vi "RESPALDO2.vi"() -> ()   [LabVIEW 2017]
uses:
  <vilib>/myRIO/Instrument Drivers/Onboard IO/PWM/typedefs/PWM Reference.ctl
  <vilib>/myRIO/Common/Instrument Driver Framework/Utilities/typedefs/myRIO Generic Hardware Reference.ctl
  <vilib>/myRIO/Common/Instrument Driver Framework/Utilities/typedefs/Hardware Version Enum.ctl
  <vilib>/myRIO/Common/Instrument Driver Framework/Utilities/typedefs/myRIO v1.0 Reference.ctl
  <vilib>/myRIO/Common/Instrument Driver Framework/Utilities/typedefs/Generic FPGA Reference.ctl
  <vilib>/myRIO/Common/Instrument Driver Framework/myRIO v1.0/PWM/typedefs/PWM Channels Enum.ctl
  <vilib>/myRIO/Instrument Drivers/Onboard IO/PWM/typedefs/PWM Configuration.ctl
  <vilib>/userdefined/High Color/nirio_resource_hc.ctl
  <vilib>/myRIO/Instrument Drivers/Onboard IO/DIO/typedefs/DIO Reference.ctl
  <vilib>/myRIO/Common/Instrument Driver Framework/myRIO v1.0/DIO/typedefs/DIO Channels List.ctl
  <vilib>/myRIO/Common/Instrument Driver Framework/myRIO v1.0/DIO/typedefs/DIO Channels Enum.ctl
  <vilib>/myRIO/Common/Instrument Driver Framework/Utilities/vis/Is FPGA Ref Available.vi
  <vilib>/myRIO/Common/Instrument Driver Framework/myRIO v1.0/DIO/vis/myRIO v1.1 Open DIO.vi
  <vilib>/myRIO/Instrument Drivers/Onboard IO/DIO/vis/Write.vi
  <vilib>/myRIO/Common/Instrument Driver Framework/myRIO v1.0/PWM/vis/myRIO v1.1 Open PWM.vi
  <vilib>/myRIO/Common/Instrument Driver Framework/myRIO v1.0/UART/vis/myRIO v1.0 Close UART.vi
  <vilib>/myRIO/Common/Instrument Driver Framework/Utilities/vis/Validate Channels.vi
  <vilib>/myRIO/Common/Instrument Driver Framework/myRIO v1.0/DIO/vis/myRIO v1.0 Reserve DIO.vi
  <vilib>/myRIO/Common/Instrument Driver Framework/myRIO v1.0/PWM/vis/myRIO v1.0 Reserve PWM.vi
  <vilib>/myRIO/Common/Instrument Driver Framework/myRIO v1.0/Resource Manager/vis/myRIO v1.0 Reserve Channel List.vi
  <vilib>/myRIO/Common/Instrument Driver Framework/myRIO v1.0/DIO/vis/myRIO v1.0 Build MUX Configuration DIO.vi
  <vilib>/myRIO/Common/Instrument Driver Framework/myRIO v1.0/PWM/vis/myRIO v1.0 Build MUX Configuration PWM.vi
  <vilib>/myRIO/Common/Instrument Driver Framework/myRIO v1.0/Resource Manager/vis/myRIO v1.0 Reserve Channel.vi
  <vilib>/myRIO/Common/Instrument Driver Framework/myRIO v1.0/Resource Manager/vis/myRIO v1.0 Unreserve Channel.vi
  <vilib>/myRIO/Common/Instrument Driver Framework/myRIO v1.0/Resource Manager/vis/myRIO v1.0 Create Configuration List.vi
  <vilib>/myRIO/Common/Instrument Driver Framework/myRIO v1.0/Resource Manager/vis/myRIO v1.0 Build Mutex Name.vi
  <vilib>/Utility/VariantDataType/GetNumericInfo.vi
  <vilib>/Utility/error.llb/Error Cluster From Error Code.vi
  <vilib>/myRIO/Common/Instrument Driver Framework/myRIO v1.0/myRIO v1.1 Open.vi
  <vilib>/myRIO/Common/Instrument Driver Framework/Utilities/vis/IO Manager.vi
  <vilib>/myRIO/Common/Instrument Driver Framework/Utilities/vis/Configuration Manager.vi
  <vilib>/myRIO/Common/Instrument Driver Framework/myRIO v1.0/Resource Manager/vis/myRIO v1.0 Configure IO.vi
  <vilib>/myRIO/Common/Instrument Driver Framework/myRIO v1.0/myRIO v1.0 Close.vi
  <vilib>/myRIO/Common/Instrument Driver Framework/myRIO v1.0/PWM/vis/myRIO v1.0 Write PWM.vi
  <vilib>/myRIO/Common/Instrument Driver Framework/myRIO v1.0/DIO/vis/myRIO v1.0 Write DIO.vi
  <vilib>/myRIO/Common/Instrument Driver Framework/Utilities/vis/FPGA Ref Manager.vi
  <vilib>/myRIO/Common/Instrument Driver Framework/myRIO v1.0/myRIO v1.0 Reset FPGA.vi
  <vilib>/myRIO/Common/Instrument Driver Framework/myRIO v1.0/IRQ/vis/myRIO v1.0 IRQ Info FGV.vi
  <vilib>/myRIO/Common/Instrument Driver Framework/myRIO v1.0/IRQ/vis/myRIO v1.0 Timer IRQ Info FGV.vi
  <vilib>/myRIO/Common/Instrument Driver Framework/myRIO v1.0/IRQ/vis/myRIO v1.0 ISR Agent.vi
  <vilib>/myRIO/Express VI/Onboard IO/PWM/PWM Express VI.xnode
  <vilib>/myRIO/Instrument Drivers/Onboard IO/PWM/vis/myRIO PWM Open.xnode
  <vilib>/myRIO/Express VI/Onboard IO/DO/DO Express VI.xnode
  <vilib>/myRIO/Instrument Drivers/Onboard IO/DIO/vis/myRIO DIO Open.xnode
  <vilib>/myRIO/Instrument Drivers/Utilities/Utilities.lvlib
  <vilib>/myRIO/Instrument Drivers/Onboard IO/PWM/PWM.lvlib
  <vilib>/myRIO/Instrument Drivers/Onboard IO/DIO/DIO.lvlib
panel:
  out "Numeric 4":dbl
  out "Numeric 3":dbl
  in  "MODO JOG":bool
  out "Numeric 2":dbl
  out "Slide 2":dbl(slide) scale=-200.0..100.0
  out "Slide":dbl(slide) scale=-200.0..100.0
  out "Numeric":dbl
  in  "control":T1(tab)
  in  "PARADA":bool
  out "ESTADO":string
  in  "?":bool
  out "MODO":string
  in  "Boolean":bool
  in  "PWM channel":tag="B/PWM0"
  in  "PWM channel 2":tag="B/PWM0"
  out "offset [%FS] 3":dbl
  in  "null offset 3":bool
  out "duty cycle [%] 3":dbl
  out "pulse width [ms] 3":dbl=1.5
  in  "position 2":dbl(slide) scale=-200.0..200.0
  in  "PWM channel 3":tag="B/PWM0"
  out "offset [%FS] 4":dbl
  in  "null offset 4":bool
  out "duty cycle [%] 4":dbl
  out "pulse width [ms] 4":dbl=1.5
  in  "position [%FS] 4":dbl(slide) scale=-200.0..200.0
  out "offset [%FS] 5":dbl
  in  "null offset 5":bool
  out "duty cycle [%] 5":dbl
  out "pulse width [ms] 5":dbl=1.5
  in  "position [%FS] 5":dbl(slide) scale=-200.0..200.0
  out "position [%FS]":dbl
  out "position [3":dbl
  out "position1":dbl
  out "ventosa":bool
  out "POSICION1":dbl
  out "POSICION2":dbl
  out "POSICION3":dbl
  in  "velocidad":dbl(knob) scale=20.0..250.0
  in  "PARADA":bool
  out "INDICADOR 2":bool
  out "INDICADOR1":bool
  in  "PARADA":bool
  in  ".":dbl(slide) scale=0.0..10.0
  in  ".":dbl(slide) scale=0.0..10.0
  out "String":string
  out "CADENA1":dbl
  out "CADENA2":dbl
  in  "Puero de servicio remoto":u16
  in  "direccion":string
  in  "PARADA":bool
  out "Datos recibidos vía TCP":cluster{dbl, dbl}(graph)
  out "offset [%FS] 2":dbl
  in  "null offset 2":bool
  out "duty cycle [%] 2":dbl
  out "pulse width [ms] 2":dbl=1.5
  in  "freq [Hz] 2":dbl=50.0
  in  "position [%FS] 3":dbl(slide) scale=-400.0..400.0
  in  "PWM channel 6":tag="B/PWM0"
  in  "PWM channel 5":tag="B/PWM0"
  in  "position [%FS] 2":dbl(slide) scale=-400.0..400.0
  in  "freq [Hz]":dbl=50.0
  out "pulse width [ms]":dbl=1.5
  out "duty cycle [%]":dbl
  in  "null offset":bool
  out "offset [%FS]":dbl
  out "offset [%FS] 6":dbl
  in  "null offset 6":bool
  out "duty cycle [%] 6":dbl
  out "pulse width [ms] 6":dbl=1.5
  in  "freq [Hz] 3":dbl=50.0
  in  "position [%FS] 6":dbl(slide) scale=-400.0..400.0
  in  "PWM channel 7":tag="B/PWM0"
  in  "VALVULA":bool
  in  "VELOCIDAD1":dbl(knob) scale=0.0..1.0
  in  "VELOCIDAD 2":dbl(knob) scale=0.0..1.0
  in  "DIRECCION1":bool
  in  "DIRECCION 2":bool
  in  "servomotores":bool
  out "V1":dbl
  out "V2":dbl
  # "BIENVENIDOS A LA\nINTERFAZ DE CONTROL ROBOT DELTA"
  # "INICIO DE PROCESO"
  # "SISTEMA DE ESTADO DE ROBOT DELTA"
  # "SERVOMOTOR1"
  # "SERVOMOTOR2"
  # "SERVOMOTOR3"
  # "VISUALIZACION DE CINTAS TRANSPORTADORAS"
  # "CINTA TRANSPORTADORA1"
  # "CINTA TRANSPORTADORA2"
  # "COMUNICACION CON EL SISTEMA DE VISION"
  # "DATOS DE COMIUNICACION"
  # "VISUALIZACION DE POSCICION"
  # "SERVOMOTOR1"
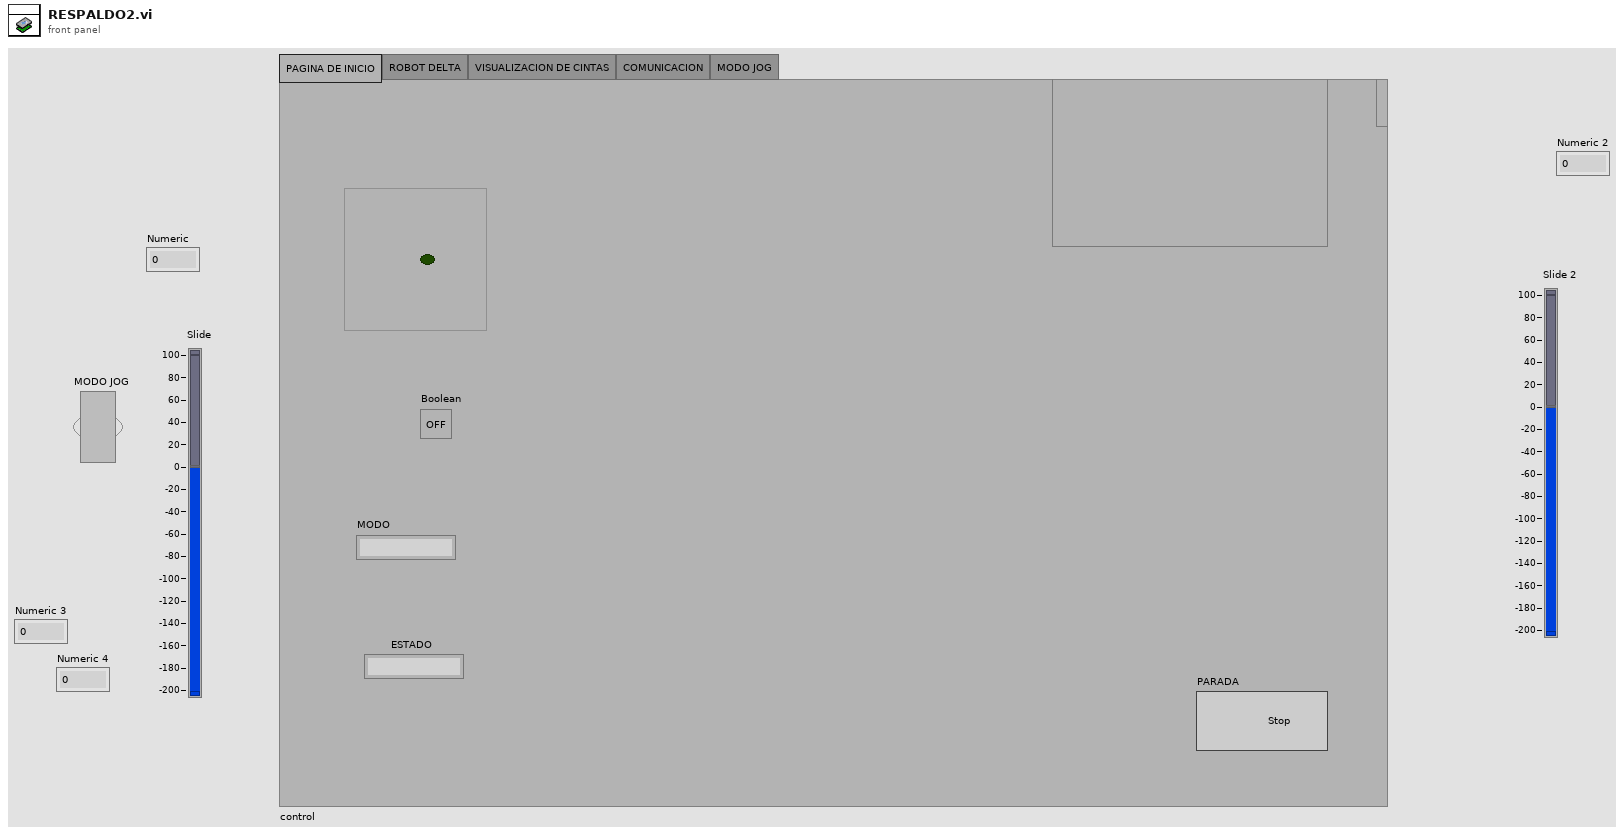
[diagram p1: front panel]
types:
  T1 = enum32{"PAGINA DE INICIO", "ROBOT DELTA", "VISUALIZACION DE CINTAS", "COMUNICACION", "MODO JOG"}
  T2 = enum16{"", "INICIO", "STOP", "DETECCION", "ESPERA", "MOVIMIENTO"}
  T3 = typedef "PWM.lvlib/PWM Reference.ctl" = cluster{"myRIO Reference":T4, "PWM Channels Enum":T8, "PWM Configuration":T9}
  T4 = typedef "myRIO Generic Hardware Reference.ctl" = cluster{"myRIO Model":T5, "myRIO Hardware Reference":T6}
  T5 = typedef "Hardware Version Enum.ctl" = enum16{"Unknown", "myRIO-1900", "myRIO-1950", "roboRIO", "NI ELVIS RIO CM"}
  T6 = typedef "myRIO v1.0 Reference.ctl" = cluster{"Generic FPGA Reference":T7, "Allow multiple opens":bool}
  T7 = typedef "Generic FPGA Reference.ctl" = refnum<k20>
  T8 = typedef "PWM Channels Enum.ctl" = enum16{"Not Connected", "C/PWM0", "C/PWM1", "A/PWM0", "A/PWM1", "A/PWM2", "B/PWM0", "B/PWM1", "B/PWM2", "PWM/PWM0", "PWM/PWM1", "PWM/PWM2", "PWM/PWM3", "PWM/PWM4", "PWM/PWM5", "PWM/PWM6", "PWM/PWM7", "PWM/PWM8", "PWM/PWM9"}
  T9 = typedef "PWM.lvlib/PWM Configuration.ctl" = cluster{"Frequency":dbl, "Duty Cycle":dbl}
  T10 = enum16{"Standard", "Buffered", "CRLF", "Immediate"}
  T11 = typedef "nirio_resource_hc.ctl" = tag
  T12 = typedef "DIO.lvlib/DIO Reference.ctl" = cluster{"myRIO Reference":T4, "DIO Channels List":T13}
  T13 = typedef "DIO Channels List.ctl" = T14[]
  T14 = typedef "DIO Channels Enum.ctl" = enum16{"Not Connected", "C/DIO0", "C/DIO1", "C/DIO2", "C/DIO3", "C/DIO4", "C/DIO5", "C/DIO6", "C/DIO7", "A/DIO0", "A/DIO1", "A/DIO2", "A/DIO3", "A/DIO4", "A/DIO5", "A/DIO6", "A/DIO7", "A/DIO8", "A/DIO9", "A/DIO10", "A/DIO11", "A/DIO12", "A/DIO13", "A/DIO14", "A/DIO15", "B/DIO0", "B/DIO1", "B/DIO2", "B/DIO3", "B/DIO4", "B/DIO5", "B/DIO6", "B/DIO7", "B/DIO8", "B/DIO9", "B/DIO10", "B/DIO11", "B/DIO12", "B/DIO13", "B/DIO14", "B/DIO15", "LED0", "LED1", "LED2", "LED3", "Button0", "DIO/DIO0", "DIO/DIO1", "DIO/DIO2", "DIO/DIO3", "DIO/DIO4", "DIO/DIO5", "DIO/DIO6", "DIO/DIO7", "DIO/DIO8", "DIO/DIO9", "SPI/CS0", "SPI/CS1", "SPI/CS2", "SPI/CS3", "LED RADIO (Green)", "LED RADIO (Red)", "LED COMM (Green)", "LED COMM (Red)", "LED MODE (Green)", "LED MODE (Red)"}
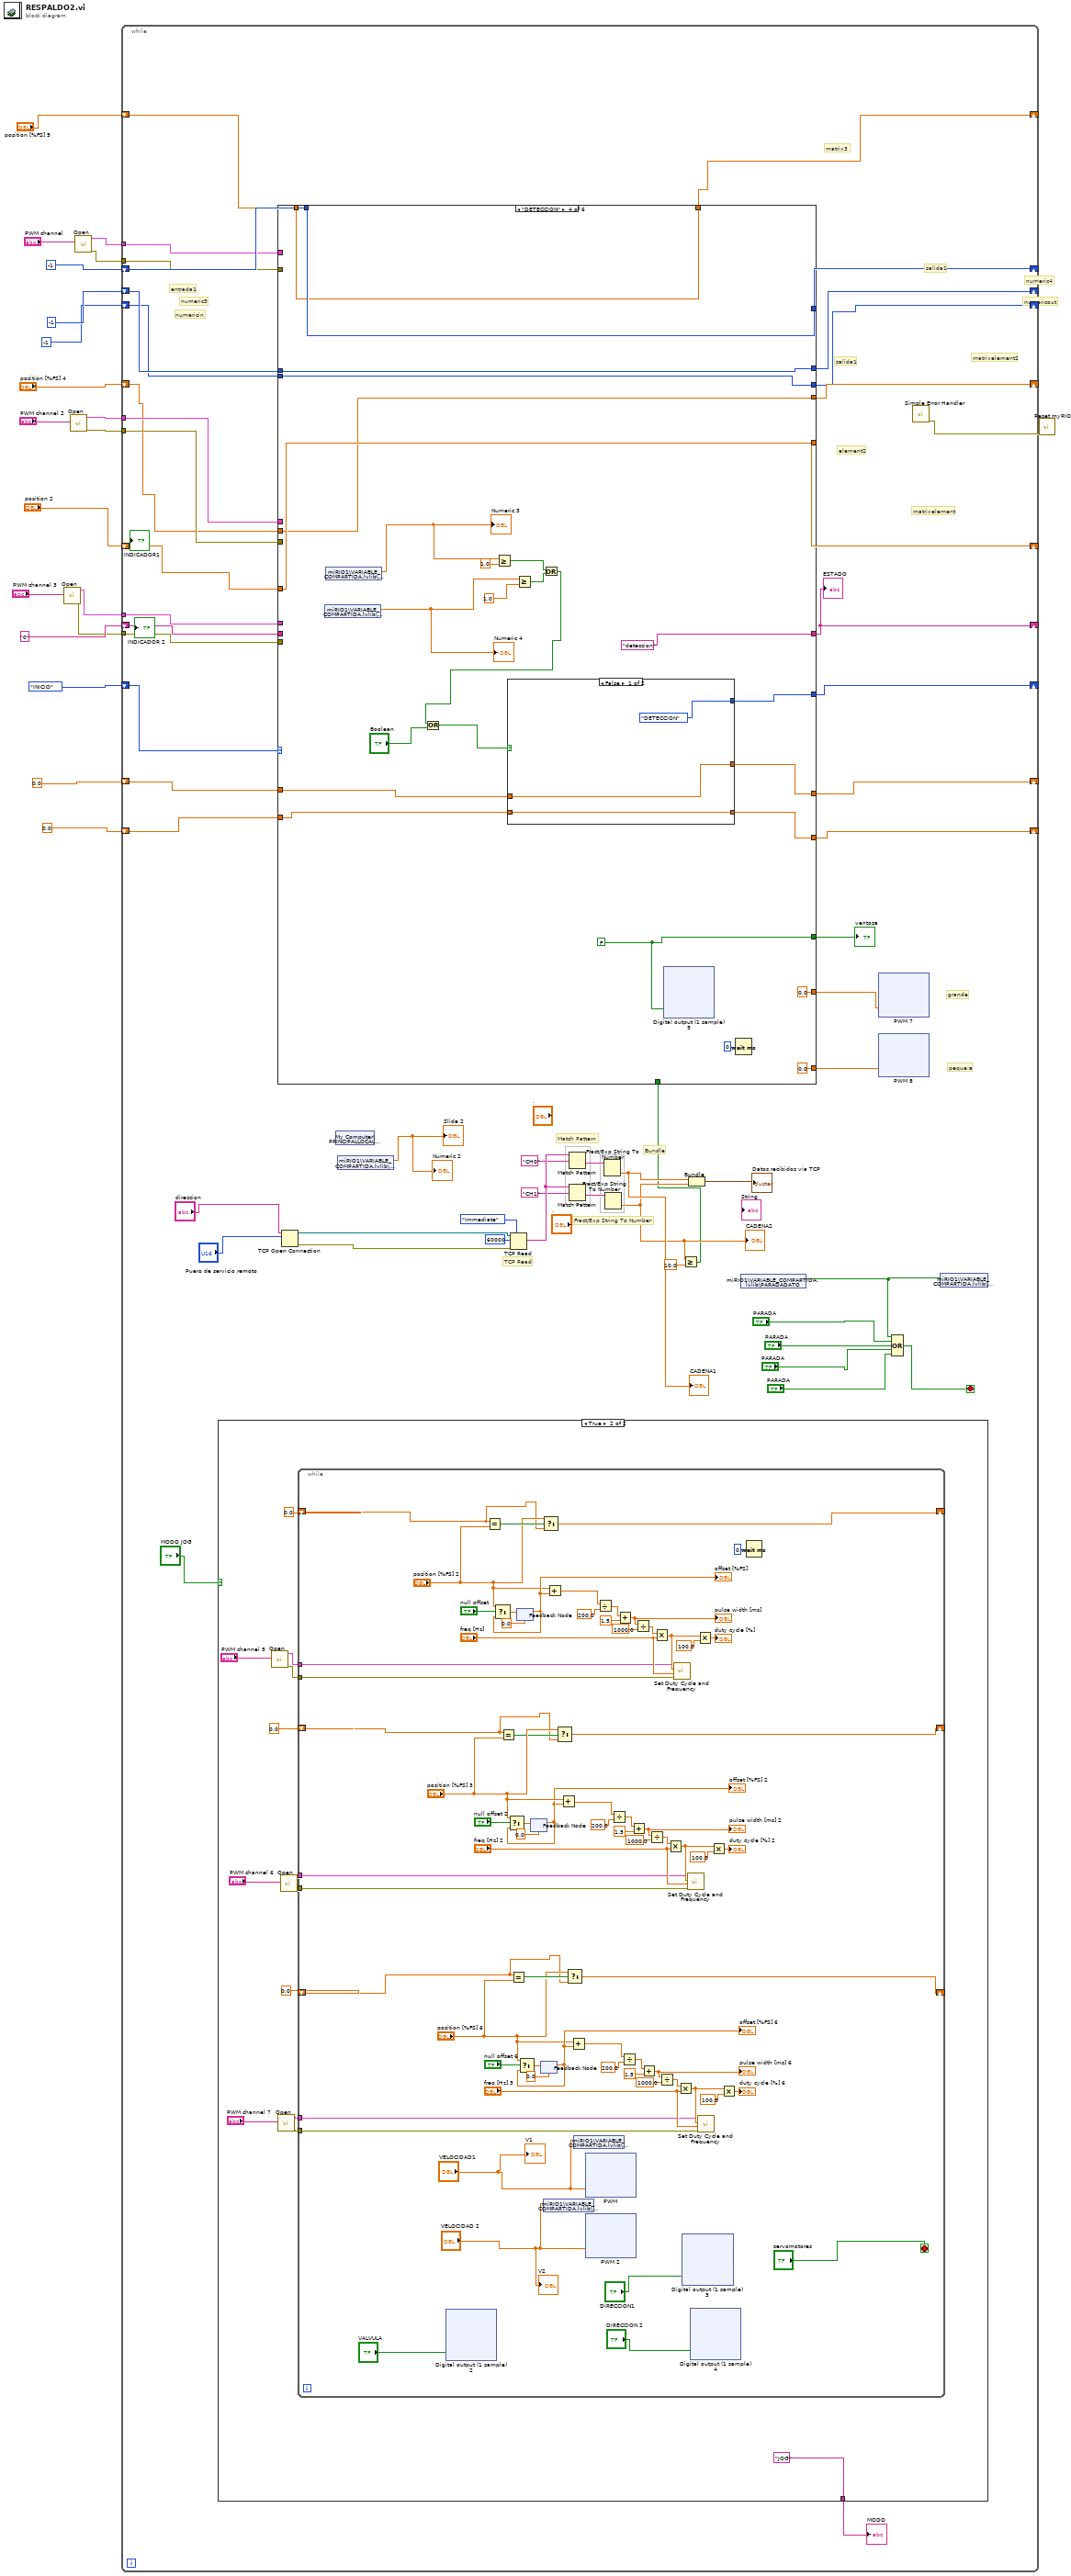
[diagram p0: block diagram]
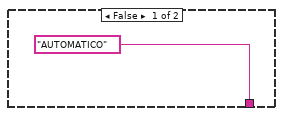
[diagram p2: hidden frame]
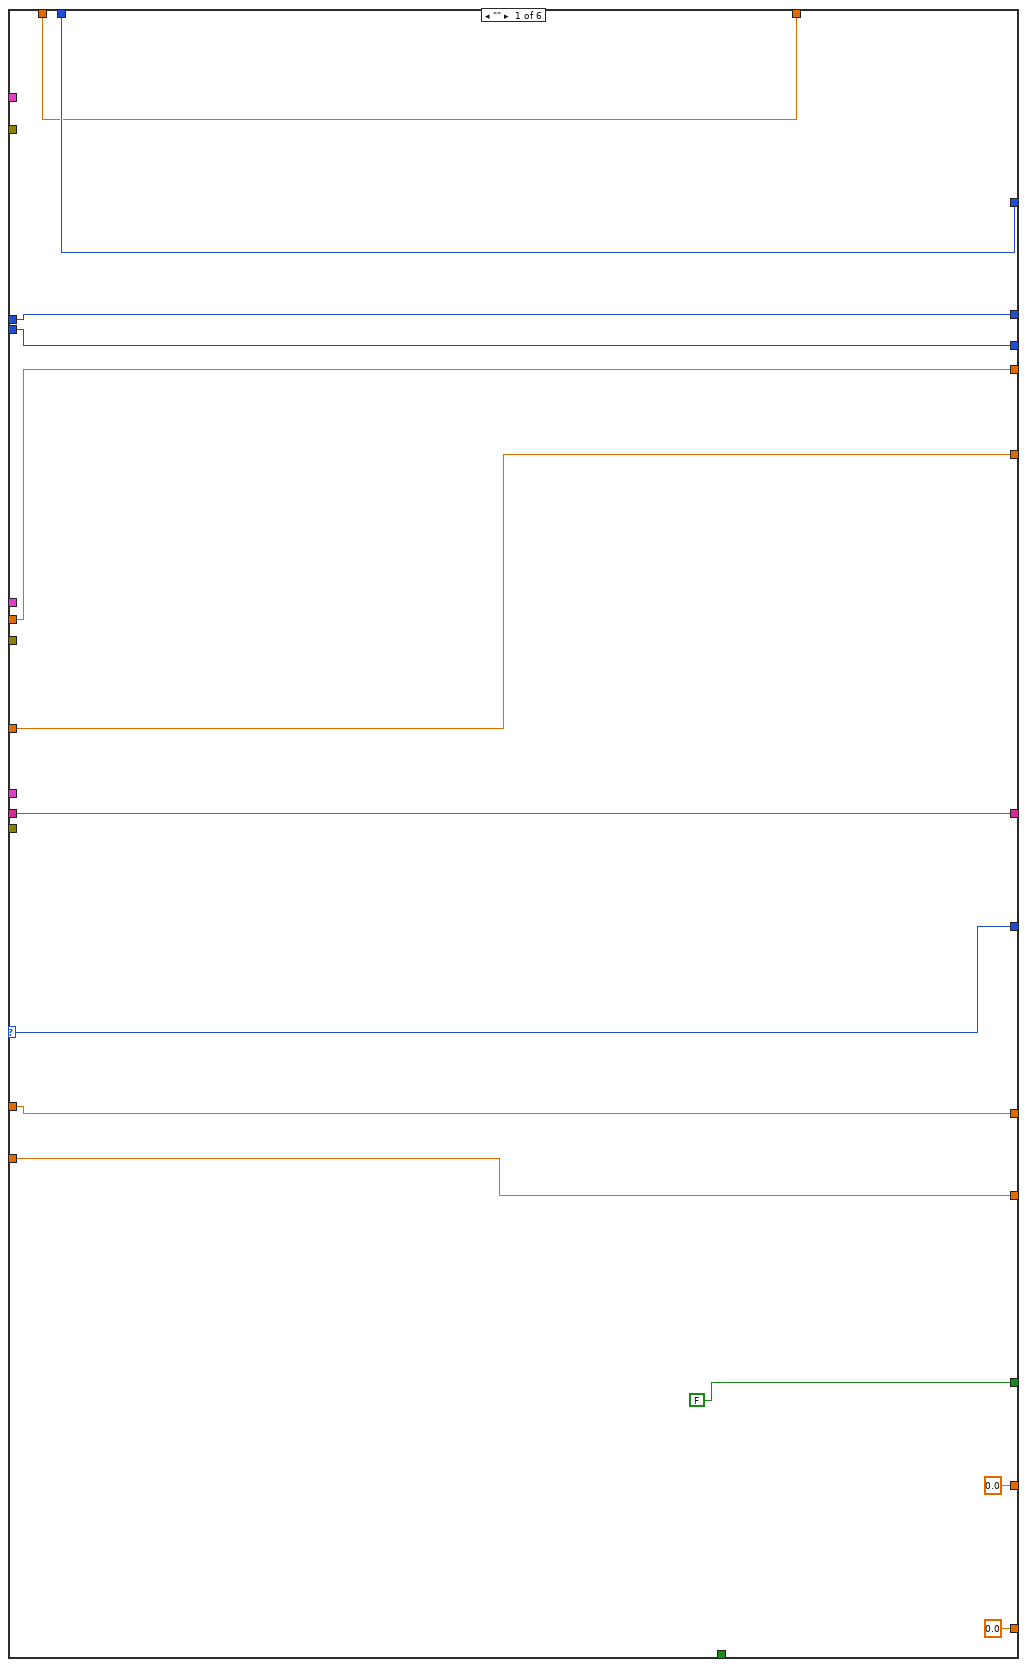
[diagram p3: hidden frame]
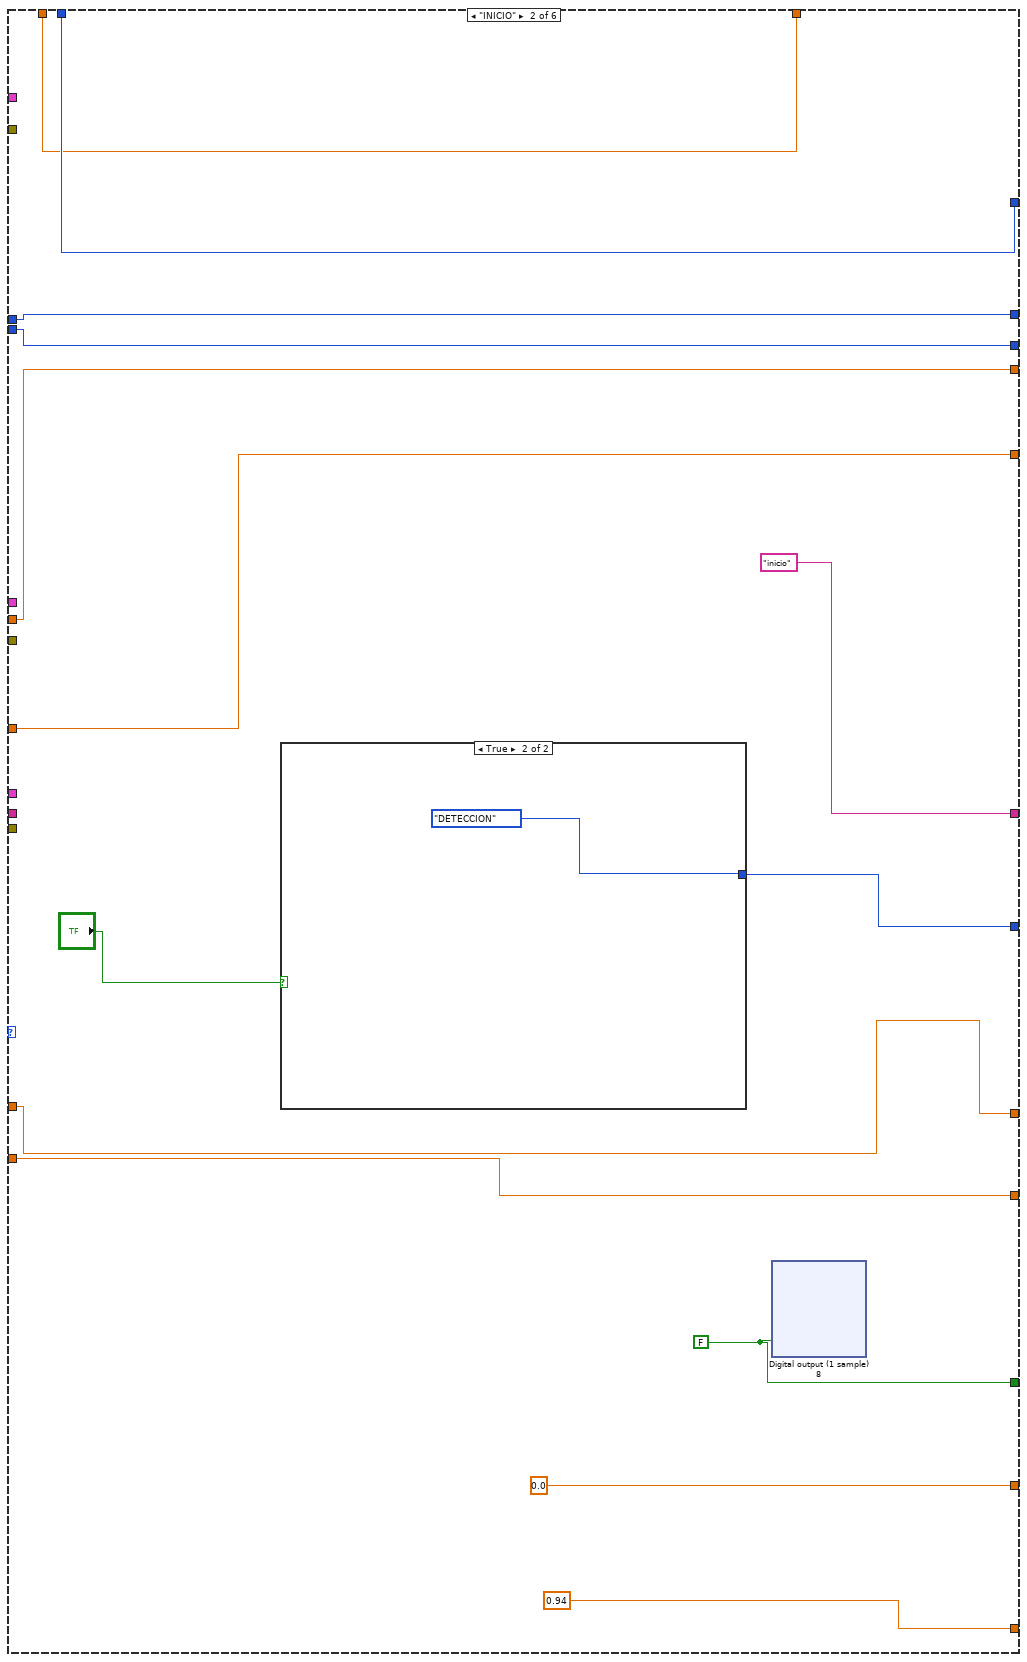
[diagram p4: hidden frame]
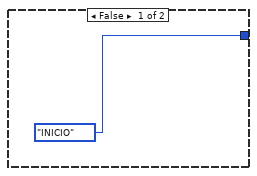
[diagram p5: hidden frame]
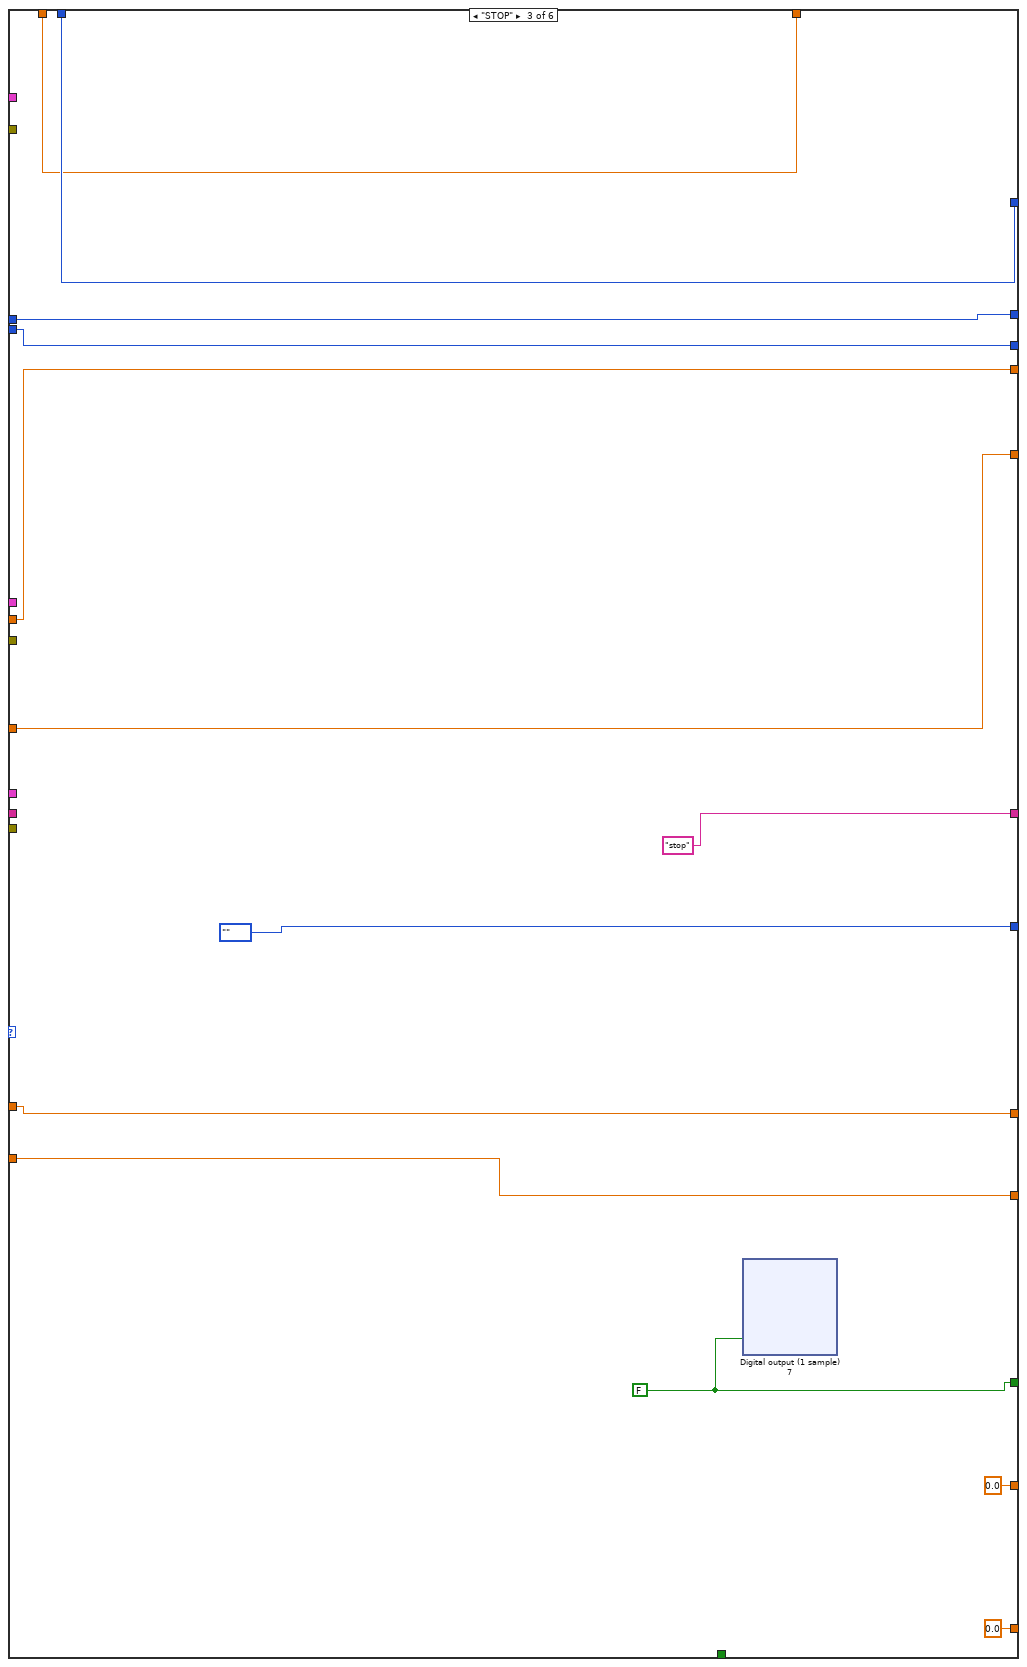
[diagram p6: hidden frame]
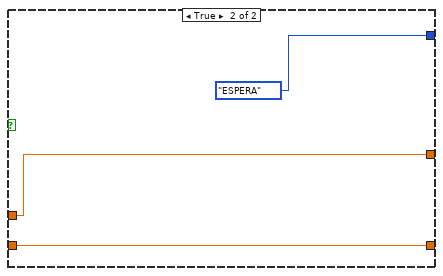
[diagram p7: hidden frame]
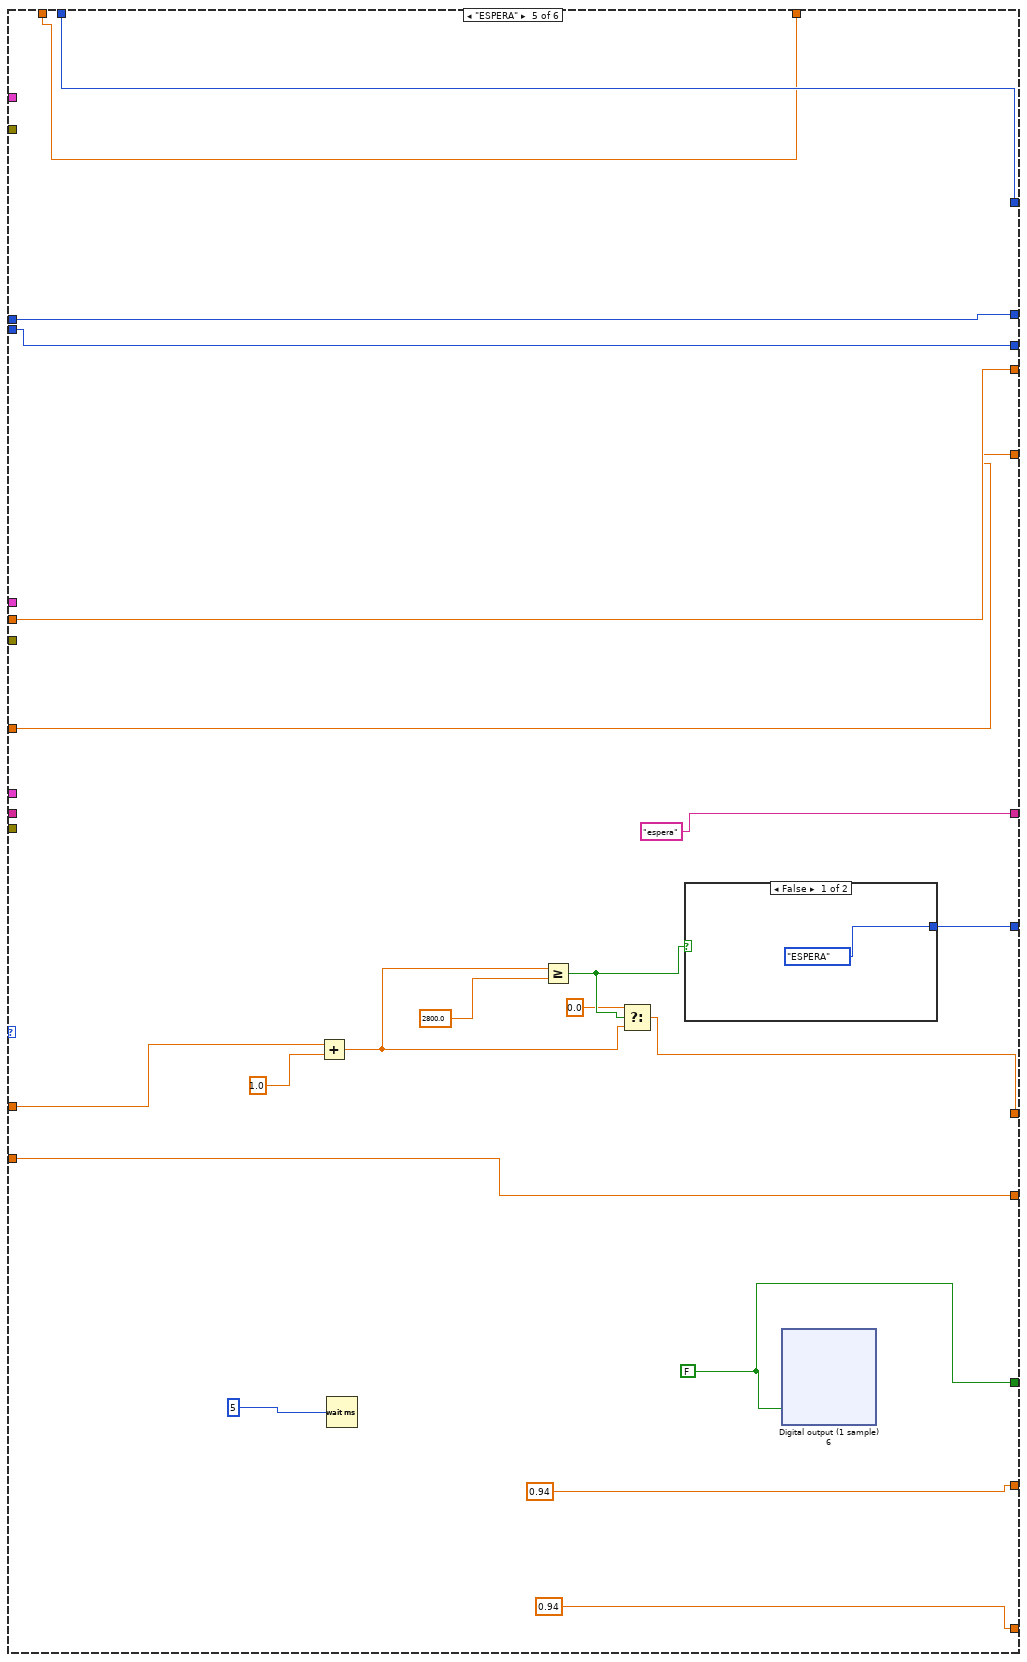
[diagram p8: hidden frame]
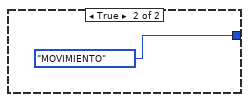
[diagram p9: hidden frame]
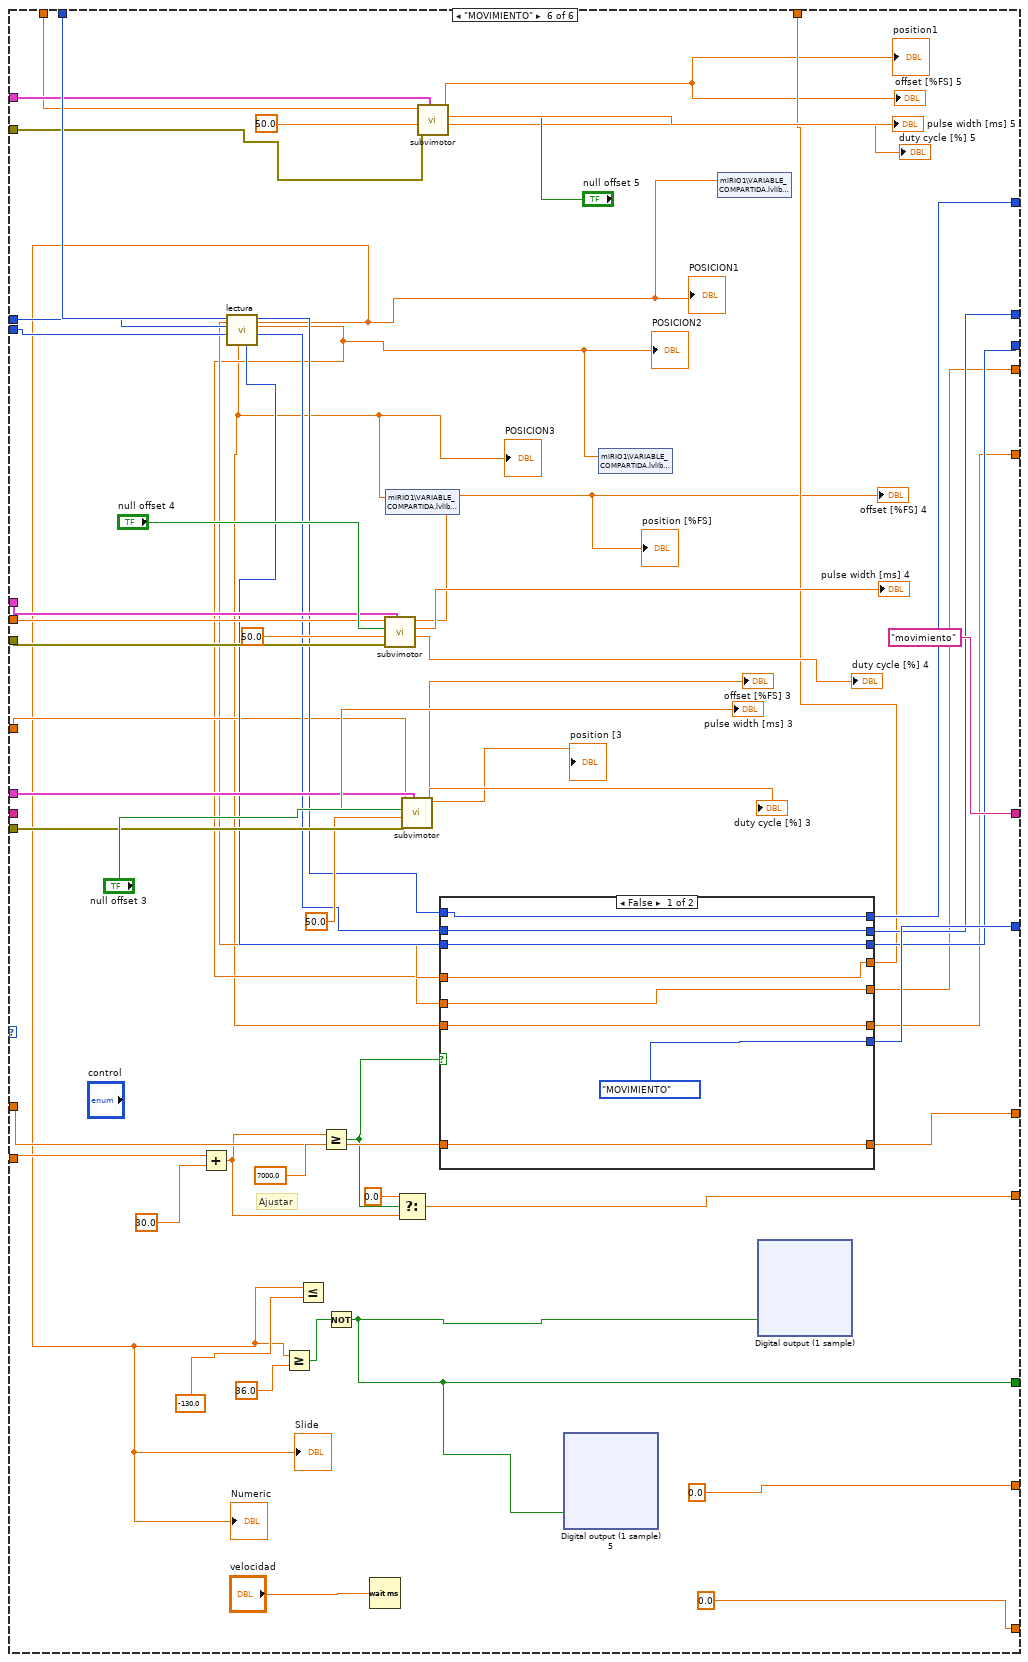
[diagram p10: hidden frame]
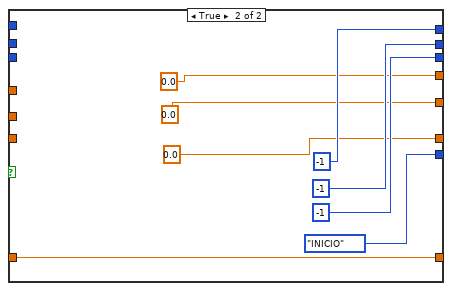
[diagram p11: hidden frame]
diagram:
  # "numericout"
  # "numeric4"
  # "salida1"
  n1 = call <vilib>:"Open.vi"("Channel Name"="PWM channel 3") -> ("error out"=w8:errorcluster, "PWM Ref Out"=w9:T3)  [unwired: 9 in]
  n2 = call <vilib>:"Open.vi"("Channel Name"="PWM channel 2") -> ("error out"=w5:errorcluster, "PWM Ref Out"=w6:T3)  [unwired: 9 in]
  n3 = call <vilib>:"Open.vi"("Channel Name"="PWM channel") -> ("error out"=w2:errorcluster, "PWM Ref Out"=w3:T3)  [unwired: 9 in]
  n4 = while {
    shift-right: [w57] -> _
    shift-left: -1 -> [w61]
    shift-right: [w55] -> _
    shift-left: -1 -> [w60]
    shift-right: [w54] -> _
    shift-left: -1 -> [w59]
    shift-right: [w58] -> _
    shift-left: "position [%FS] 5" -> [w50]
    shift-right: [w56] -> _
    shift-left: "position [%FS] 4" -> [w62]
    shift-right: [w53] -> _
    shift-left: "position 2" -> [w65]
    shift-right: [w73] -> _
    shift-left: T2."INICIO" -> [w74]
    shift-right: [w72] -> _
    shift-left: 0.0 -> [w71]
    shift-right: [w70] -> _
    shift-left: 0.0 -> [w49]
    shift-right: [w69] -> _
    shift-left: "0" ("String") -> [w68]
    tunnel: w9 -> [w67]
    tunnel: w8 -> [w66]
    tunnel: w6 -> [w64]
    tunnel: w5 -> [w63]
    tunnel: w3 -> [w52]
    tunnel: w2 -> [w51]
    stop <- w24 stop-if-true
    # "grande"
    # "peque;a"
    # "matrixelement2"
    # "matrixelement"
    # "Bundle"
    # "TCP Read"
    # "Fract/Exp String To Number"
    # "Match Pattern"
    # "element2"
    # "salida1"
    # "matrix3"
    # "numericin"
    # "numeric3"
    # "entrada1"
    n5 = case shown="True" "MODO JOG" {
      tunnel: ["AUTOMATICO" ("MODO") "JOG" ("MODO")] -> w26
      frame False {
      }
      frame True {
        n6 = call <vilib>:"Open.vi"("Channel Name"="PWM channel 5") -> ("error out"=w156:errorcluster, "PWM Ref Out"=w157:T3)  [unwired: 9 in]
        n7 = call <vilib>:"Open.vi"("Channel Name"="PWM channel 7") -> ("error out"=w150:errorcluster, "PWM Ref Out"=w151:T3)  [unwired: 9 in]
        n8 = call <vilib>:"Open.vi"("Channel Name"="PWM channel 6") -> ("error out"=w153:errorcluster, "PWM Ref Out"=w154:T3)  [unwired: 9 in]
        n9 = while {
          tunnel: w157 -> [w210]
          tunnel: w156 -> [w209]
          shift-right: [w208] -> _
          shift-left: 0.0 ("position [%FS] 2") -> [w207]
          shift-right: [w188] -> _
          shift-left: 0.0 ("position [%FS] 3") -> [w189]
          tunnel: w154 -> [w187]
          tunnel: w153 -> [w186]
          shift-right: [w167] -> _
          shift-left: 0.0 ("position [%FS] 6") -> [w168]
          tunnel: w151 -> [w166]
          tunnel: w150 -> [w165]
          stop <- "servomotores" stop-if-true
          n10 = xnode "Digital output (1 sample) 2"("B/DIO2 (Pin 15)"="VALVULA") -> ()  [unwired: 1 in, 1 out]
          n11 = Equal?(x=w207, y="position [%FS] 2") -> (x = y?=w212:bool)
          n12 = Equal?(x=w189, y="position [%FS] 3") -> (x = y?=w205:bool)
          n13 = Equal?(x=w168, y="position [%FS] 6") -> (x = y?=w170:bool)
          n14 = feedback #1(0.0 ("position [%FS]")) -> (w218:dbl)
          "offset [%FS]" <- w218
          n15 = Select(t="position [%FS] 2", s="null offset", f=w218) -> (s? t:f=w220:dbl)
          n16 = feedback-in #1(w220) -> ()
          n17 = feedback #2(0.0 ("position [%FS]")) -> (w199:dbl)
          "offset [%FS] 2" <- w199
          n18 = Select(t="position [%FS] 3", s="null offset 2", f=w199) -> (s? t:f=w197:dbl)
          n19 = feedback-in #2(w197) -> ()
          n20 = feedback #3(0.0 ("position [%FS]")) -> (w176:dbl)
          "offset [%FS] 6" <- w176
          n21 = Select(t="position [%FS] 6", s="null offset 6", f=w176) -> (s? t:f=w178:dbl)
          n22 = feedback-in #3(w178) -> ()
          n23 = Select(t="position [%FS] 2", s=w212, f=w207) -> (s? t:f=w208:dbl)
          n24 = shared-variable "miRIO1\\VARIABLE_COMPARTIDA.lvlib\\MOTOR2"("VELOCIDAD 2") -> ()  [unwired: 1 in, 1 out]
          n25 = Add(x="position [%FS] 2", y=w218) -> (x+y=w219:dbl)
          n26 = Select(t="position [%FS] 3", s=w205, f=w189) -> (s? t:f=w188:dbl)
          n27 = Add(x="position [%FS] 3", y=w199) -> (x+y=w198:dbl)
          n28 = Select(t="position [%FS] 6", s=w170, f=w168) -> (s? t:f=w167:dbl)
          n29 = Add(x="position [%FS] 6", y=w176) -> (x+y=w177:dbl)
          n30 = shared-variable "miRIO1\\VARIABLE_COMPARTIDA.lvlib\\MOTOR1"("VELOCIDAD1") -> ()  [unwired: 1 in, 1 out]
          n31 = xnode "PWM"("Duty Cycle"="VELOCIDAD1") -> ()  [unwired: 1 in, 1 out]
          n32 = xnode "PWM 2"("Duty Cycle"="VELOCIDAD 2") -> ()  [unwired: 1 in, 1 out]
          n33 = Divide(x=w219, y=200.0) -> (x/y=w226:dbl)
          n34 = Divide(x=w198, y=200.0) -> (x/y=w191:dbl)
          n35 = Add(x=w226, y=1.5) -> (x+y=w224:dbl)
          "pulse width [ms]" <- w224
          n36 = Divide(x=w177, y=200.0) -> (x/y=w184:dbl)
          n37 = Add(x=w191, y=1.5) -> (x+y=w193:dbl)
          "pulse width [ms] 2" <- w193
          n38 = Divide(x=w224, y=1000.0) -> (x/y=w217:dbl)
          n39 = Add(x=w184, y=1.5) -> (x+y=w182:dbl)
          "pulse width [ms] 6" <- w182
          n40 = Divide(x=w193, y=1000.0) -> (x/y=w200:dbl)
          n41 = Multiply(x=w217, y="freq [Hz]") -> (x*y=w214:dbl)
          n42 = Divide(x=w182, y=1000.0) -> (x/y=w175:dbl)
          n43 = Multiply(x=w200, y="freq [Hz] 2") -> (x*y=w203:dbl)
          n44 = call <vilib>:"Set Duty Cycle and Frequency.vi"("error in (no error)"=w209, "Frequency [Hz]"="freq [Hz]", "Duty Cycle"=w214, "PWM Ref In"=w210) -> ()  [unwired: 5 in, 2 out]
          n45 = Multiply(x=w175, y="freq [Hz] 3") -> (x*y=w172:dbl)
          n46 = xnode "Digital output (1 sample) 3"("B/DIO0 (Pin 11)"="DIRECCION1") -> ()  [unwired: 1 in, 1 out]
          n47 = call <vilib>:"Set Duty Cycle and Frequency.vi"("error in (no error)"=w186, "Frequency [Hz]"="freq [Hz] 2", "Duty Cycle"=w203, "PWM Ref In"=w187) -> ()  [unwired: 5 in, 2 out]
          n48 = xnode "Digital output (1 sample) 4"("B/DIO1 (Pin 13)"="DIRECCION 2") -> ()  [unwired: 1 in, 1 out]
          n49 = Multiply(x=w214, y=100.0) -> (x*y=→"duty cycle [%]":dbl)
          n50 = call <vilib>:"Set Duty Cycle and Frequency.vi"("error in (no error)"=w165, "Frequency [Hz]"="freq [Hz] 3", "Duty Cycle"=w172, "PWM Ref In"=w166) -> ()  [unwired: 5 in, 2 out]
          n51 = Multiply(x=w203, y=100.0) -> (x*y=→"duty cycle [%] 2":dbl)
          n52 = Multiply(x=w172, y=100.0) -> (x*y=→"duty cycle [%] 6":dbl)
          n53 = Wait (ms)(milliseconds to wait=u32 0) -> ()  [unwired: 1 out]
          "V1" <- "VELOCIDAD1"
          "V2" <- "VELOCIDAD 2"
        }
      }
    }
    "MODO" <- w26
    n54 = TCP Open Connection(address="direccion", remote port or service name="Puero de servicio remoto") -> (connection ID=w48:refnum<k5>, error out=w47:errorcluster)  [unwired: 3 in]
    n55 = shared-variable "My Computer\\PRINCIPALLOCAL1.lvlib\\POS1"() -> ()  [unwired: 1 in, 2 out]
    n56 = shared-variable "miRIO1\\VARIABLE_COMPARTIDA.lvlib\\POSICION1"() -> (→"Slide 2" →"Numeric 2":dbl)  [unwired: 1 in, 1 out]
    n57 = TCP Read(connection ID=w48, bytes to read=60000, error in (no error)=w47, 7:T10."Immediate" ("mode (standard)")) -> (data out=w44:string)  [unwired: 1 in, 2 out]
    n58 = Match Pattern(string=w44, regular expression="CH0") -> (after substring=w46:string)  [unwired: 1 in, 3 out]
    n59 = Match Pattern(string=w44, regular expression="CH1") -> (after substring=w45:string)  [unwired: 1 in, 3 out]
    n60 = Fract/Exp String To Number(string=w46) -> (number=w42:dbl)  [unwired: 3 in, 1 out]
    "CADENA1" <- w42
    n61 = Fract/Exp String To Number(string=w45) -> (number=w37:dbl)  [unwired: 3 in, 1 out]
    "CADENA2" <- w37
    n62 = Greater Or Equal?(x=w37, y=10.0) -> (x >= y?=w35:bool)
    n63 = case shown="\"DETECCION\"" w74 {
      selector: w74 -> [w416 _ _ _ _ _]
      tunnel: [w416 w430 T2."" w540 w598 w693] -> w73
      tunnel: [w415 w429 w479 w539 w593 w692] -> w72
      tunnel: w71 -> [w415 w429 w479 w538 w600 w691]
      tunnel: [w414 w428 w478 w537 w597 w686] -> w70
      tunnel: w49 -> [w414 w428 w478 w536 w597 w653]
      tunnel: [w413 "inicio" ("String") "stop" ("String") "deteccion" ("String") "espera" ("String") "movimiento" ("String")] -> w69
      tunnel: w68 -> [w413 _ _ _ _ _]
      tunnel: w67 -> [_ _ _ _ _ w682]
      tunnel: w66 -> [_ _ _ _ _ w681]
      tunnel: w65 -> [w408 w421 w471 w530 w586 w652]
      tunnel: w64 -> [_ _ _ _ _ w676]
      tunnel: w63 -> [_ _ _ _ _ w675]
      tunnel: w62 -> [w409 w422 w472 w529 w587 w673]
      tunnel: w61 -> [w412 w426 w476 w534 w589 w672]
      tunnel: w60 -> [w411 w425 w475 w533 w591 w671]
      tunnel: w59 -> [w410 w424 w474 w532 w590 w670]
      tunnel: [w407 w423 w473 w531 w588 w656] -> w58
      tunnel: [w412 w426 w476 w534 w589 w661] -> w57
      tunnel: [w409 w422 w472 w529 w587 w655] -> w56
      tunnel: [w411 w425 w475 w533 w591 w659] -> w55
      tunnel: [w410 w424 w474 w532 w590 w657] -> w54
      tunnel: [w408 w421 w471 w530 w586 w654] -> w53
      tunnel: w52 -> [_ _ _ _ _ w666]
      tunnel: w51 -> [_ _ _ _ _ w665]
      tunnel: w50 -> [w407 w423 w473 w531 w588 w663]
      tunnel: w35 -> [_ _ _ _ _ _]
      tunnel: [FALSE w419 w470 w528 w585 w650] -> w25
      tunnel: [0.0 ("Duty Cycle") 0.94 ("Duty Cycle") 0.0 ("Duty Cycle") 0.0 ("Duty Cycle") 0.94 ("Duty Cycle") 0.0 ("Duty Cycle")] -> w22
      tunnel: [0.0 ("Duty Cycle") 0.0 ("Duty Cycle") 0.0 ("Duty Cycle") 0.0 ("Duty Cycle") 0.94 ("Duty Cycle") 0.0 ("Duty Cycle")] -> w21
      frame "" {
      }
      frame "INICIO" {
        w419 = FALSE ("B/DIO2 (Pin 15)")
        n64 = case shown="True" "?" {
          tunnel: [T2."INICIO" T2."DETECCION"] -> w430
          frame False {
          }
          frame True {
          }
        }
        n65 = xnode "Digital output (1 sample) 8"("B/DIO2 (Pin 15)"=w419) -> ()  [unwired: 1 in, 1 out]
      }
      frame "STOP" {
        w470 = FALSE ("B/DIO2 (Pin 15)")
        n66 = xnode "Digital output (1 sample) 7"("B/DIO2 (Pin 15)"=w470) -> ()  [unwired: 1 in, 1 out]
      }
      frame "DETECCION" {
        w528 = FALSE ("B/DIO2 (Pin 15)")
        n67 = shared-variable "miRIO1\\VARIABLE_COMPARTIDA.lvlib\\POSICION2"() -> (w527:dbl)  [unwired: 1 in, 1 out]
        "Numeric 4" <- w527
        n68 = shared-variable "miRIO1\\VARIABLE_COMPARTIDA.lvlib\\POSICION1"() -> (w526:dbl)  [unwired: 1 in, 1 out]
        "Numeric 3" <- w526
        n69 = Greater Or Equal?(x=w526, y=1.0) -> (x >= y?=w523:bool)
        n70 = Greater Or Equal?(x=w527, y=1.0) -> (x >= y?=w522:bool)
        n71 = Or(x=w523, y=w522) -> (x .or. y?=w519:bool)
        n72 = Or(x=w519, y="Boolean") -> (x .or. y?=w520:bool)
        n73 = case shown="False" w520 {
          tunnel: [T2."DETECCION" T2."ESPERA"] -> w540
          tunnel: [w577 w580] -> w539
          tunnel: w538 -> [w577 w580]
          tunnel: [w576 w579] -> w537
          tunnel: w536 -> [w576 w579]
          frame False {
          }
          frame True {
          }
        }
        n74 = xnode "Digital output (1 sample) 9"("B/DIO2 (Pin 15)"=w528) -> ()  [unwired: 1 in, 1 out]
        n75 = Wait (ms)(milliseconds to wait=u32 0) -> ()  [unwired: 1 out]
      }
      frame "ESPERA" {
        w585 = FALSE ("B/DIO2 (Pin 15)")
        n76 = Add(x=w600, y=1.0) -> (x+y=w594:dbl)
        n77 = Wait (ms)(milliseconds to wait=u32 5) -> ()  [unwired: 1 out]
        n78 = Greater Or Equal?(x=w594, y=2800.0) -> (x >= y?=w595:bool)
        n79 = Select(t=0.0, s=w595, f=w594) -> (s? t:f=w593:dbl)
        n80 = case shown="False" w595 {
          tunnel: [T2."ESPERA" T2."MOVIMIENTO"] -> w598
          frame False {
          }
          frame True {
          }
        }
        n81 = xnode "Digital output (1 sample) 6"("B/DIO2 (Pin 15)"=w585) -> ()  [unwired: 1 in, 1 out]
      }
      frame "MOVIMIENTO" {
        # "Ajustar"
        n82 = Add(x=w653, y=30.0) -> (x+y=w687:dbl)
        n83 = call "lectura.vi"("Numeric in"=w670, "Numeric 3"=w671, "entrada1"=w672) -> ("Numeric 4"=w660:i32, "Real Matrix Element 2"=w643:dbl, "salida1"=w662:i32, "Numeric out"=w658:i32, "Real Matrix Element 3"=w644:dbl, "Real Matrix Element"=w642:dbl)  [unwired: 3 in]
        "POSICION1" <- w644
        "POSICION2" <- w643
        "POSICION3" <- w642
        "Slide" <- w644
        "Numeric" <- w644
        n84 = Greater Or Equal?(x=w644, y=36.0) -> (x >= y?=w648:bool)
        n85 = Less Or Equal?(x=w644, y=-130.0) -> ()  [unwired: 1 out]
        n86 = Greater Or Equal?(x=w687, y=7000.0) -> (x >= y?=w689:bool)
        n87 = Not(x=w648) -> (.not. x?=w650:bool)
        n88 = Wait (ms)(milliseconds to wait="velocidad") -> ()  [unwired: 1 out]
        n89 = call "subvimotor.vi"("PWM Ref Out"=w676, "error in (no error)"=w675, "freq [Hz] 3"=50.0, "null offset 3"="null offset 4", "position [%FS] 3"=w673) -> ("Numeric"=→"duty cycle [%] 4":dbl, "Numeric 2"=→"pulse width [ms] 4":dbl, "position [%FS]"=→"offset [%FS] 4" →"position [%FS]":dbl)  [unwired: 4 in]
        n90 = shared-variable "miRIO1\\VARIABLE_COMPARTIDA.lvlib\\ZPOS"(w642) -> ()  [unwired: 1 in, 1 out]
        n91 = Select(t=0.0, s=w689, f=w687) -> (s? t:f=w686:dbl)
        n92 = call "subvimotor.vi"("PWM Ref Out"=w682, "error in (no error)"=w681, "freq [Hz] 3"=50.0, "null offset 3"="null offset 3", "position [%FS] 3"=w652) -> ("Numeric"=→"duty cycle [%] 3":dbl, "Numeric 2"=→"pulse width [ms] 3":dbl, "position [%FS]"=→"offset [%FS] 3" →"position [3":dbl)  [unwired: 4 in]
        n93 = call "subvimotor.vi"("PWM Ref Out"=w666, "error in (no error)"=w665, "freq [Hz] 3"=50.0, "null offset 3"="null offset 5", "position [%FS] 3"=w663) -> ("Numeric"=→"duty cycle [%] 5":dbl, "Numeric 2"=→"pulse width [ms] 5":dbl, "position [%FS]"=→"offset [%FS] 5" →"position1":dbl)  [unwired: 4 in]
        n94 = case shown="False" w689 {
          tunnel: [T2."MOVIMIENTO" T2."INICIO"] -> w693
          tunnel: [w772 w780] -> w692
          tunnel: w691 -> [w772 w780]
          tunnel: w662 -> [w771 _]
          tunnel: [w771 -1] -> w661
          tunnel: w660 -> [w770 _]
          tunnel: [w770 -1] -> w659
          tunnel: w658 -> [w769 _]
          tunnel: [w769 -1] -> w657
          tunnel: w644 -> [w768 _]
          tunnel: [w768 0.0 ("t")] -> w656
          tunnel: w643 -> [w767 _]
          tunnel: [w767 0.0 ("t")] -> w655
          tunnel: w642 -> [w766 _]
          tunnel: [w766 0.0 ("t")] -> w654
          frame False {
          }
          frame True {
          }
        }
        n95 = xnode "Digital output (1 sample) 5"("B/DIO2 (Pin 15)"=w650) -> ()  [unwired: 1 in, 1 out]
        n96 = shared-variable "miRIO1\\VARIABLE_COMPARTIDA.lvlib\\YPOS"(w643) -> ()  [unwired: 1 in, 1 out]
        n97 = shared-variable "miRIO1\\VARIABLE_COMPARTIDA.lvlib\\XPOS"(w644) -> ()  [unwired: 1 in, 1 out]
        n98 = xnode "Digital output (1 sample)"("A/DIO1 (Pin 13)"=w650) -> ()  [unwired: 1 in, 1 out]
      }
    }
    "ESTADO" <- w69
    "ventosa" <- w25
    n99 = Bundle(w42, w37) -> (→"Datos recibidos vía TCP":cluster{dbl, dbl})  [unwired: 1 in]
    n100 = shared-variable "miRIO1\\VARIABLE_COMPARTIDA.lvlib\\PARADADATO"() -> (w23:bool)  [unwired: 1 in, 1 out]
    n101 = xnode "PWM 7"("Duty Cycle"=w21) -> ()  [unwired: 1 in, 1 out]
    n102 = xnode "PWM 8"("Duty Cycle"=w22) -> ()  [unwired: 1 in, 1 out]
    n103 = Compound Arithmetic op=OR(w23, "PARADA", "PARADA", "PARADA", "PARADA") -> (w24:bool)
    n104 = shared-variable "miRIO1\\VARIABLE_COMPARTIDA.lvlib\\PARADA"(w23) -> ()  [unwired: 1 in, 1 out]
  }
  n105 = call <vilib>:"Simple Error Handler.vi"() -> ("error out"=w20:errorcluster)  [unwired: 5 in, 4 out]
  n106 = call <vilib>:"Reset myRIO.vi"("error in (no error)"=w20) -> ()  [unwired: 10 in, 1 out]
